vi "Keithley 2450 DC Block Timed with Stim Trigger.vi"() -> ()   [LabVIEW 2020]
uses:
  <vilib>/DAQmx/write.llb/DAQmx Write (Analog Wfm 1Chan NSamp).vi
  <vilib>/DAQmx/create/channels.llb/DAQmx Create Channel (AO-Voltage-Basic).vi
  <vilib>/DAQmx/configure/timing.llb/DAQmx Timing (Use Waveform).vi
  <vilib>/DAQmx/miscellaneous.llb/DAQmx Fill In Error Info.vi
  <instrlib>/Keithley 2450/Public/Data/Read (Multiple Points).vi
  <vilib>/measure/NI_MABase.lvlib
  <vilib>/Analysis/NI_AALBase.lvlib
  <instrlib>/Keithley 2450/Keithley 2450.lvlib
panel:
  in  "Source Mode":enum16{"Voltage", "Current"}(ring)=enum."Current"
  in  "VISA resource name":refnum<visa-resource-name>
  in  "Compliance\nVoltage (V)":dbl=210.0
  in  "stop":bool
  out "Waveform Graph":waveform(dbl)(graph)
  in  "NI DAQ Trigger Channel":tag
  in  "Block\nDuration (s)":dbl=10.0 min=0.0 step=0.001
  in  "Block\nAmplitude (mU)":dbl=-1.0
  in  "Pulse-to-Block\nDelay (ms)":dbl=0.1 min=0.0 step=1.0
  in  "Min # Pulses\nBefore Block":u8=4 step=1
  in  "Pulse\nFrequency (Hz)":dbl=1.0 min=0.01 max=50.0
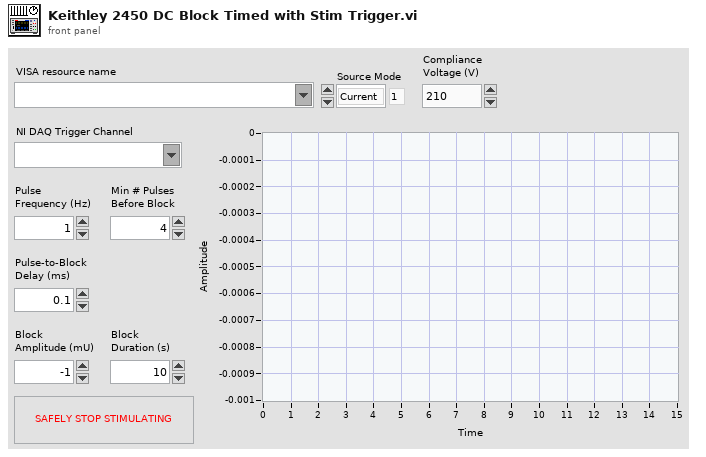
[diagram p1: front panel]
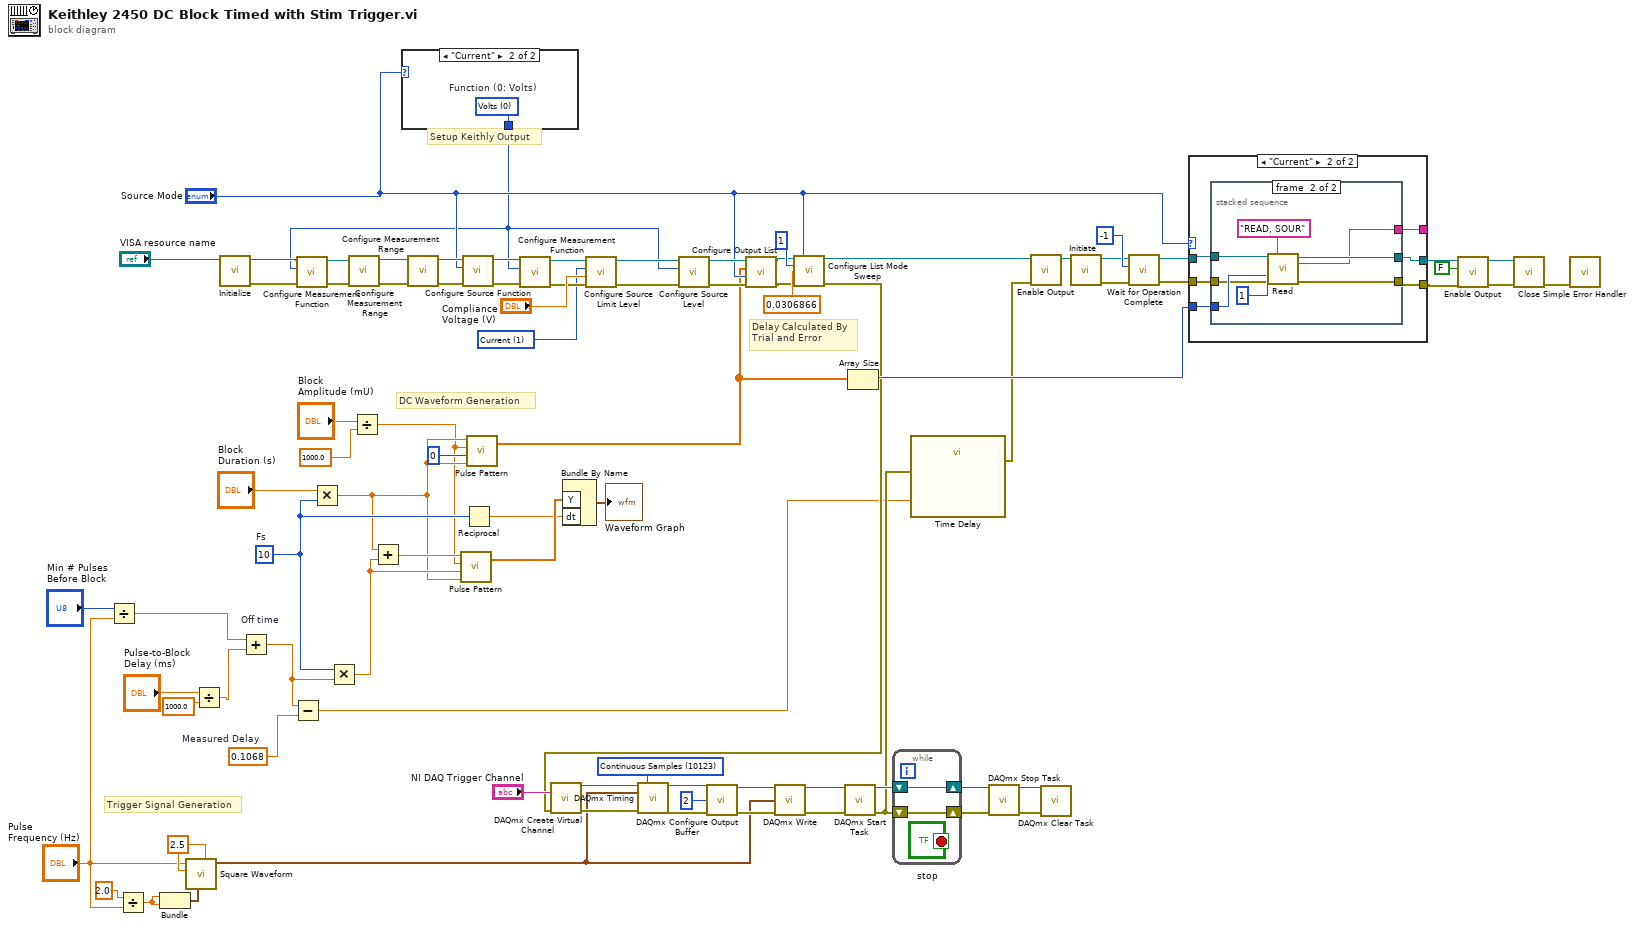
[diagram p0: block diagram]
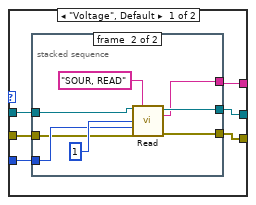
[diagram p2: hidden frame]
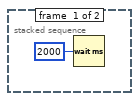
[diagram p3: hidden frame]
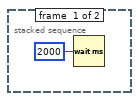
[diagram p4: hidden frame]
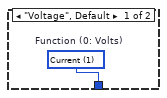
[diagram p5: hidden frame]
diagram:
  w20 = u16 1 items=["Volts", "Current"] ("Function (0: Volts)")
  w51 = 0.1068  # Measured Delay
  w67 = 10123 items=["Finite Samples"=10178, "Continuous Samples"=10123, "Hardware Timed Single Point"=12522] ("sample mode")
  w71 = 10  # Fs
  w85 = 2.5 ("amplitude")
  # "Delay Calculated By\nTrial and Error"
  # "Setup Keithly Output"
  # "Trigger Signal Generation"
  # "DC Waveform Generation"
  n1 = Divide(x="Min # Pulses\nBefore Block", y="Pulse\nFrequency (Hz)") -> (x/y=w79:dbl)
  n2 = Divide(x=2.0, y="Pulse\nFrequency (Hz)") -> (x/y=w82:dbl)
  n3 = Bundle(w82, w82) -> (w83:cluster{dbl, dbl})  [unwired: 1 in]
  n4 = call <vilib>:"Square Waveform.vi"("offset"=w85, "sampling info"=w83, "amplitude"=w85, "frequency"="Pulse\nFrequency (Hz)") -> ("signal out"=w61:waveform(dbl))  [unwired: 6 in, 1 out]
  n5 = Divide(x="Pulse-to-Block\nDelay (ms)", y=1000.0) -> (x/y=w53:dbl)
  n6 = call <instrlib>:"Initialize.vi"("VISA resource name"="VISA resource name") -> ("error out"=w41:errorcluster, "VISA resource name out"=w39:refnum<visa-resource-name>)  [unwired: 9 in]
  n7 = Add "Off time"(x=w79, y=w53) -> (x+y=w3:dbl)
  n8 = Subtract(x=w3, y=w51) -> (x-y=w2:dbl)
  n9 = Multiply(x="Block\nDuration (s)", y=w71) -> (x*y=w10:dbl)
  n10 = Multiply(x=w71, y=w3) -> (x*y=w76:dbl)
  n11 = Divide(x="Block\nAmplitude (mU)", y=1000.0) -> (x/y=w9:dbl)
  n12 = Add(x=w10, y=w76) -> (x+y=w75:dbl)
  n13 = case shown="\"Current\"" "Source Mode" {
    tunnel: [w86 w87] -> w1
    frame "Voltage", Default {
      w86 = u16 1 items=["Volts", "Current", "Resistance"]  # Function (0: Volts)
    }
    frame "Current" {
      w87 = u16 0 items=["Volts", "Current", "Resistance"]  # Function (0: Volts)
    }
  }
  n14 = call <instrlib>:"Configure Measurement Function.vi"("error in (no error)"=w41, "Function (0: Volts)"=w1, "VISA resource name"=w39) -> ("error out"=w40:errorcluster, "VISA resource name out"=w38:refnum<visa-resource-name>)  [unwired: 7 in]
  n15 = call <instrlib>:"Configure Measurement Range.vi"("error in (no error)"=w40, "VISA resource name"=w38) -> ("error out"=w47:errorcluster, "VISA resource name out"=w46:refnum<visa-resource-name>)  [unwired: 8 in]
  n16 = call <instrlib>:"Configure Measurement Range.vi"("error in (no error)"=w47, "VISA resource name"=w46) -> ("error out"=w37:errorcluster, "VISA resource name out"=w36:refnum<visa-resource-name>)  [unwired: 8 in]
  n17 = call <vilib>:"Pulse Pattern.vi"("width"=w10, "delay"=w76, "amplitude"=w9, "samples"=w75) -> ("Pulse Pattern"=w52:dbl[])  [unwired: 1 out]
  n18 = call <instrlib>:"Configure Source Function.vi"("error in (no error)"=w37, "Function (0: Volts)"="Source Mode", "VISA resource name"=w36) -> ("error out"=w28:errorcluster, "VISA resource name out"=w31:refnum<visa-resource-name>)  [unwired: 7 in]
  n19 = Reciprocal(x=w71) -> (1/x=w50:dbl)
  n20 = call <vilib>:"Pulse Pattern.vi"("width"=w10, "delay"=0, "amplitude"=w9, "samples"=w10) -> ("Pulse Pattern"=w14:dbl[])  [unwired: 1 out]
  n21 = call <instrlib>:"Configure Measurement Function.vi"("error in (no error)"=w28, "Function (0: Volts)"=w1, "VISA resource name"=w31) -> ("error out"=w29:errorcluster, "VISA resource name out"=w30:refnum<visa-resource-name>)  [unwired: 7 in]
  n22 = Bundle By Name("Y"=w52, "dt"=w50) -> (→"Waveform Graph":waveform(dbl))  [unwired: 1 in]
  n23 = call <instrlib>:"Configure Source Limit Level.vi"("error in (no error)"=w29, "Source Limit (1.0)"="Compliance\nVoltage (V)", "Function (0: Volts)"=w20, "VISA resource name"=w30) -> ("error out"=w16:errorcluster, "VISA resource name out"=w17:refnum<visa-resource-name>)  [unwired: 6 in]
  n24 = call <instrlib>:"Configure Source Level.vi"("error in (no error)"=w16, "Function (0: Volts)"=w1, "VISA resource name"=w17) -> ("error out"=w24:errorcluster, "VISA resource name out"=w25:refnum<visa-resource-name>)  [unwired: 7 in]
  n25 = call <instrlib>:"Configure Output List.vi"("error in (no error)"=w24, "Source Mode  (0: Voltage)"="Source Mode", "Output List"=w14, "VISA resource name"=w25) -> ("error out"=w7:errorcluster, "VISA resource name out"=w8:refnum<visa-resource-name>)  [unwired: 6 in]
  n26 = call <instrlib>:"Configure List Mode Sweep.vi"("VISA resource name"=w8, "Source Mode  (0: Voltage)"="Source Mode", "Start Index"=u32 1, "Delay (0)"=0.0306866, "error in (no error)"=w7) -> ("VISA resource name out"=w5:refnum<visa-resource-name>, "error out"=w11:errorcluster)  [unwired: 9 in]
  n27 = call-poly <vilib>:"DAQmx Create Virtual Channel.vi"("physical channels"="NI DAQ Trigger Channel", "error in"=w11) -> ("task out"=w69:refnum<k21>, "error out"=w68:errorcluster)  [unwired: 12 in]
  n28 = call-poly <vilib>:"DAQmx Timing.vi"("task/channels in"=w69, "sample mode"=w67, "waveform"=w61, "error in"=w68) -> ("task out"=w65:refnum<k21>, "error out"=w64:errorcluster)  [unwired: 10 in]
  n29 = call <vilib>:"DAQmx Configure Output Buffer.vi"("task/channels in"=w65, "buffer size (in samples per channel)"=u32 2, "error in"=w64) -> ("task out"=w63:refnum<k21>, "error out"=w62:errorcluster)  [unwired: 11 in]
  n30 = call-poly <vilib>:"DAQmx Write.vi"("task/channels in"=w63, "data"=w61, "error in"=w62) -> ("task out"=w60:refnum<k21>, "error out"=w56:errorcluster)  [unwired: 10 in, 1 out]
  n31 = call <vilib>:"DAQmx Start Task.vi"("task/channels in"=w60, "error in"=w56) -> ("task out"=w58:refnum<k21>, "error out"=w12:errorcluster)  [unwired: 12 in]
  n32 = Array Size(array=w14) -> (size(s)=w13:i32)
  n33 = while {
    shift-right: [w89] -> w59
    shift-left: w58 -> [w89]
    shift-right: [w88] -> w57
    shift-left: w12 -> [w88]
    stop <- "stop" stop-if-true
  }
  n34 = call "Time Delay"("error in (no error)"=w12, "Delay Time (s)"=w2) -> ("error out"=w4:errorcluster)  [unwired: 9 in]
  n35 = call <vilib>:"DAQmx Stop Task.vi"("task/channels in"=w59, "error in"=w57) -> ("task out"=w74:refnum<k21>, "error out"=w73:errorcluster)  [unwired: 12 in]
  n36 = call <instrlib>:"Enable Output.vi"("error in (no error)"=w4, "VISA resource name"=w5) -> ("VISA resource name out"=w6:refnum<visa-resource-name>)  [unwired: 8 in, 1 out]
  n37 = call <vilib>:"DAQmx Clear Task.vi"("task in"=w74, "error in"=w73) -> ()  [unwired: 13 in, 1 out]
  n38 = call <instrlib>:"Initiate.vi"("VISA resource name"=w6) -> ("error out"=w33:errorcluster, "VISA resource name out"=w15:refnum<visa-resource-name>)  [unwired: 9 in]
  n39 = call <instrlib>:"Wait for Operation Complete.vi"("error in (no error)"=w33, "Timeout (10000 ms)"=-1, "VISA resource name"=w15) -> ("error out"=w27:errorcluster, "VISA resource name out"=w22:refnum<visa-resource-name>)  [unwired: 7 in]
  n40 = case shown="\"Current\"" "Source Mode" {
    tunnel: [w96 w110] -> w19
    tunnel: [w95 w109] -> w18
    tunnel: w13 -> [w94 w111]
    tunnel: [w93 w108] -> _
    tunnel: w27 -> [w92 w107]
    tunnel: w22 -> [w91 w106]
    frame "Voltage", Default {
      n41 = stacked-sequence {
        tunnel: [_ w105] -> w96
        tunnel: [_ w104] -> w95
        tunnel: [_ w102] -> w93
        tunnel: w94 -> [_ w100]
        tunnel: w92 -> [_ w99]
        tunnel: w91 -> [_ w98]
        frame #0 {
          n42 = Wait (ms)(milliseconds to wait=u32 2000) -> ()  [unwired: 1 out]
        }
        frame #1 {
          n43 = call-poly <instrlib>:"Read.vi"("VISA resource name"=w98, "Buffer Elements"="SOUR, READ", "Start Index (1)"=1, "End Index (1)"=w100, "error in (no error)"=w99) -> ("VISA resource name out"=w105:refnum<visa-resource-name>, "Data out"=w102:string, "error out"=w104:errorcluster)  [unwired: 8 in]
        }
      }
    }
    frame "Current" {
      n44 = stacked-sequence {
        tunnel: [_ w120] -> w110
        tunnel: [_ w119] -> w109
        tunnel: [_ w117] -> w108
        tunnel: w111 -> [_ w115]
        tunnel: w107 -> [_ w114]
        tunnel: w106 -> [_ w113]
        frame #0 {
          n45 = Wait (ms)(milliseconds to wait=u32 2000) -> ()  [unwired: 1 out]
        }
        frame #1 {
          n46 = call-poly <instrlib>:"Read.vi"("VISA resource name"=w113, "Buffer Elements"="READ, SOUR", "Start Index (1)"=1, "End Index (1)"=w115, "error in (no error)"=w114) -> ("VISA resource name out"=w120:refnum<visa-resource-name>, "Data out"=w117:string, "error out"=w119:errorcluster)  [unwired: 8 in]
        }
      }
    }
  }
  n47 = call <instrlib>:"Enable Output.vi"("error in (no error)"=w18, "Enable Output (T: Enable)"=FALSE, "VISA resource name"=w19) -> ("error out"=w43:errorcluster, "VISA resource name out"=w42:refnum<visa-resource-name>)  [unwired: 7 in]
  n48 = call <instrlib>:"Close.vi"("error in (no error)"=w43, "VISA resource name"=w42) -> ("error out"=w44:errorcluster)  [unwired: 9 in]
  n49 = call <vilib>:"Simple Error Handler.vi"("error in (no error)"=w44) -> ()  [unwired: 4 in, 5 out]
